vi "Main Controls.vi"() -> ()   [LabVIEW 2024]
panel:
  out "connection information":path
  out "System Number":string
  out "Idle Time":timestamp
  in  "Remove Positions":bool
  in  "Transfer Board":bool
  in  "System Summary":bool
  in  "Add Positions":bool
  in  "Exit":bool
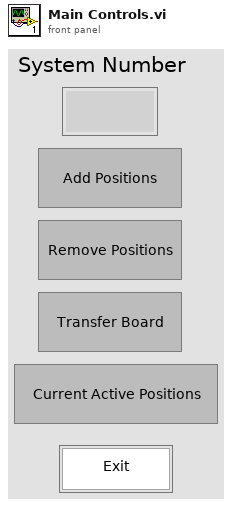
[diagram p1: front panel]
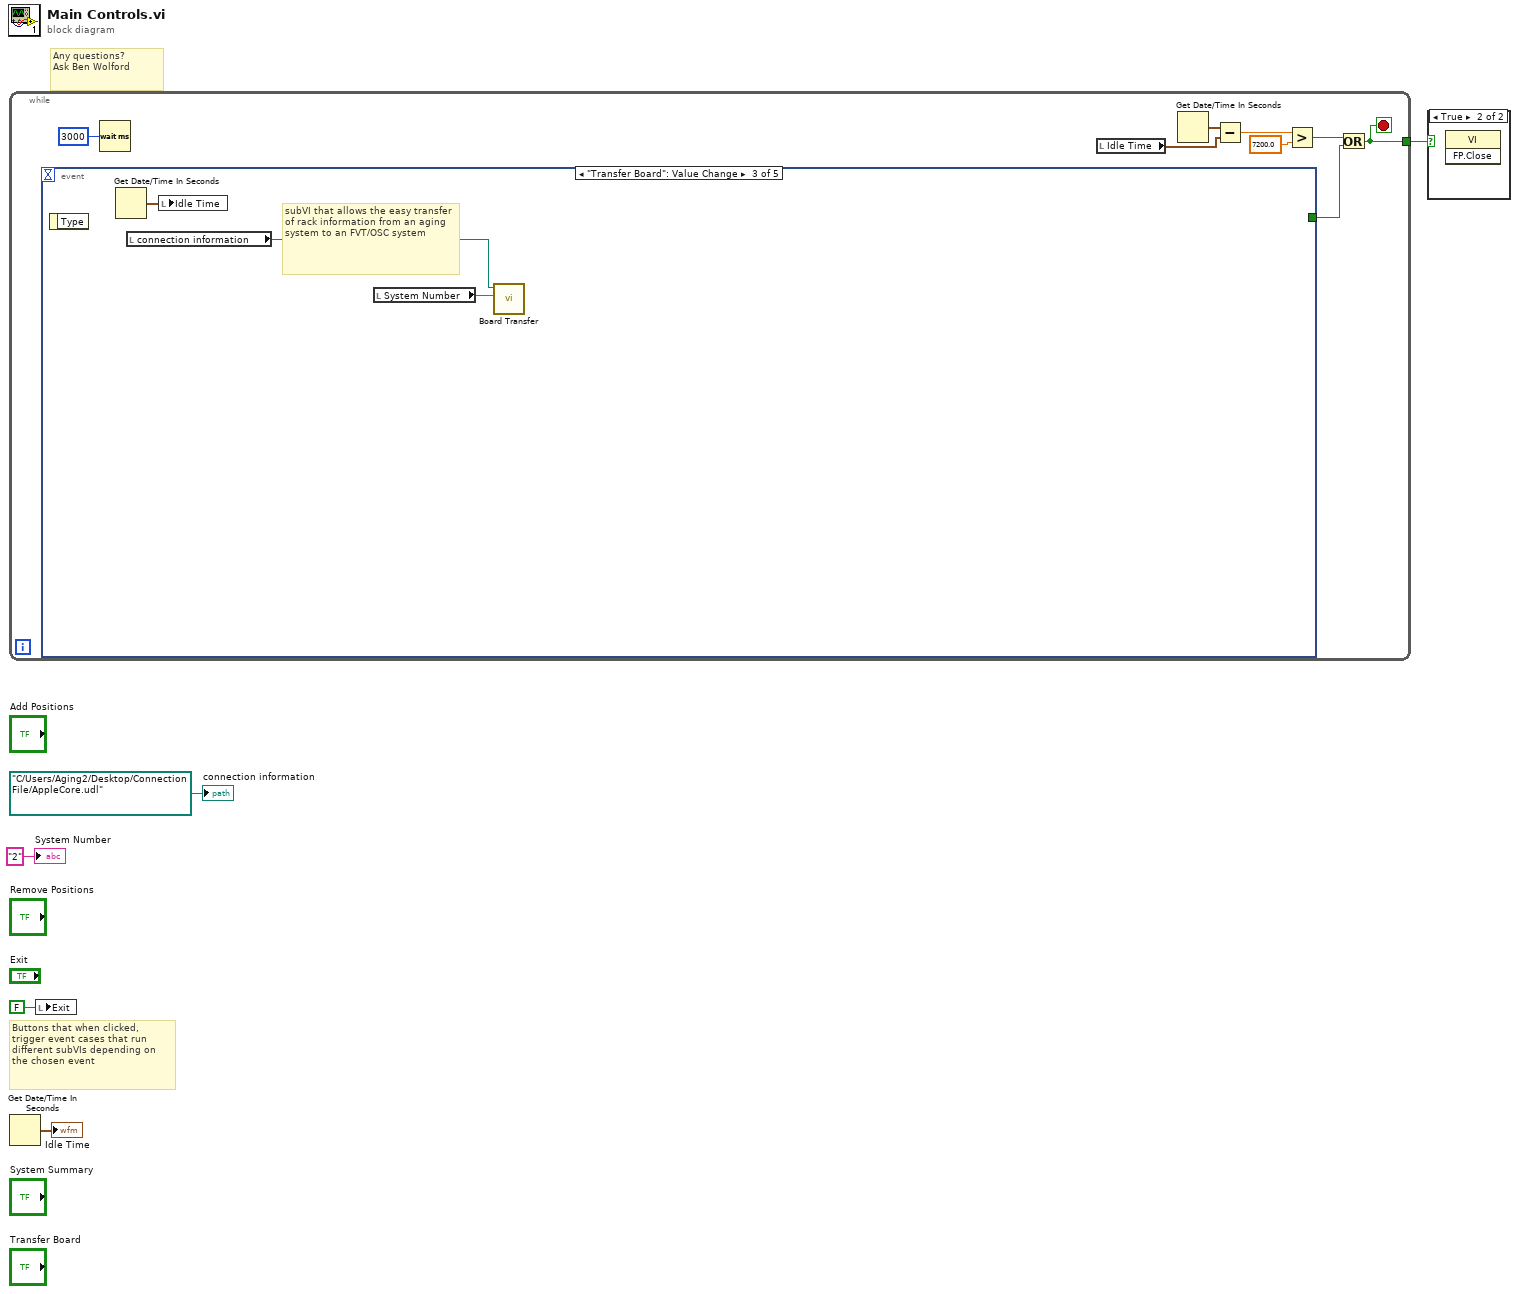
[diagram p0: block diagram]
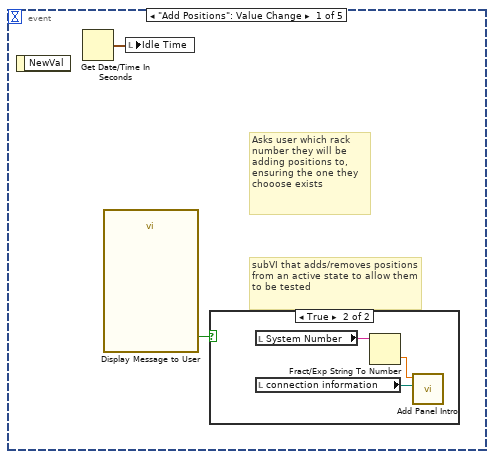
[diagram p3: hidden frame]
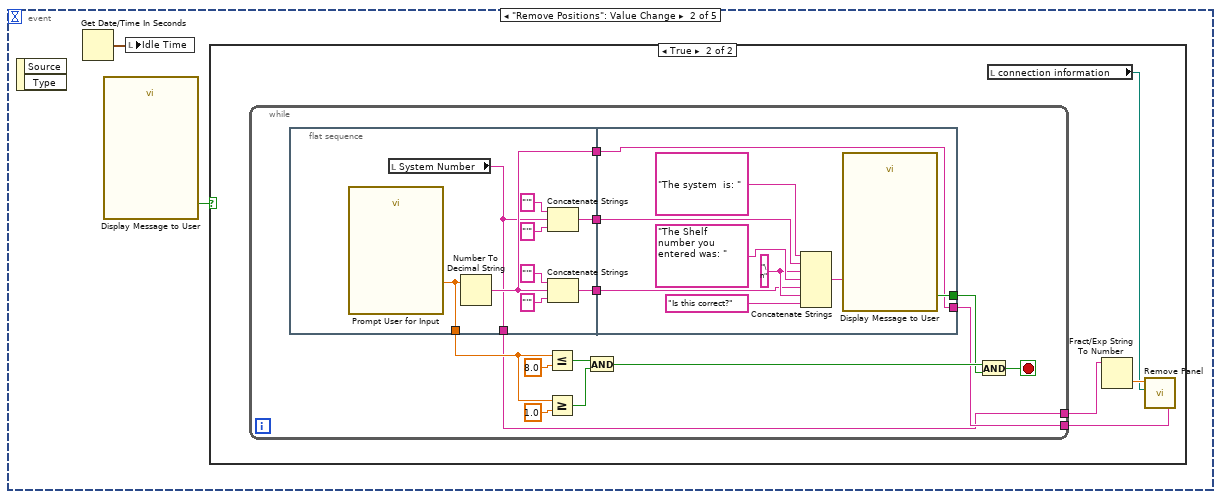
[diagram p5: hidden frame]
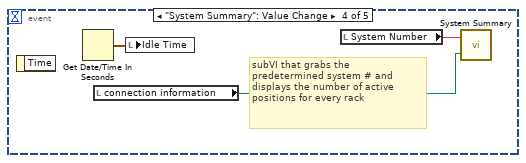
[diagram p7: hidden frame]
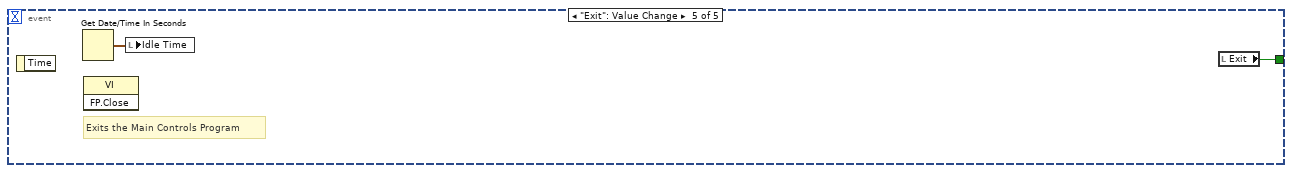
[diagram p8: hidden frame]
diagram:
  # "Buttons that when clicked, trigger event cases that run different subVIs depending on the chosen event"
  # "Any questions?\nAsk Ben Wolford"
  n1 = while {
    tunnel: [w6] -> w1
    stop <- w6 stop-if-true
    n2 = event shown="[2] \"Transfer Board\": Value Change" {
      selector: _ -> [_ _ _ _ _]
      dyn-events: _ -> [_ _ _ _ _]
      timeout: _ -> [_ _ _ _ _]
      tunnel: [_ _ _ _ w63] -> w12
      event "Add Positions": Value Change {
        # "Asks user which rack number they will be adding positions to, ensuring the one they chooose exists"
        # "subVI that adds/removes positions from an active state to allow them to be tested"
        n3 = event-data() -> ()  [unwired: 1 in, 1 out]
        n4 = Get Date/Time In Seconds() -> (seconds since 1Jan1904=w14:timestamp)
        n5 = call "Display Message to User"() -> ("Yes"=w15:bool)  [unwired: 10 in, 1 out]
        n6 = local write "Idle Time"(w14) -> ()
        n7 = case shown="True" w15 {
          frame False {
          }
          frame True {
            n8 = local read "System Number"() -> (w18:string)
            n9 = local read "connection information"() -> (w16:path)
            n10 = Fract/Exp String To Number(string=w18) -> (number=w17:dbl)  [unwired: 3 in, 1 out]
            n11 = call "Add Panel Intro.vi"("connection information"=w16, "System Number"=w17) -> ()  [unwired: 10 in]
          }
        }
      }
      event "Remove Positions": Value Change {
        n12 = event-data() -> ()  [unwired: 1 in, 2 out]
        n13 = Get Date/Time In Seconds() -> (seconds since 1Jan1904=w19:timestamp)
        n14 = call "Display Message to User"() -> ("Yes"=w20:bool)  [unwired: 10 in, 1 out]
        n15 = local write "Idle Time"(w19) -> ()
        n16 = case shown="True" w20 {
          frame False {
          }
          frame True {
            n17 = while {
              tunnel: [w26] -> w23
              tunnel: [w27] -> w24
              stop <- w29 stop-if-true
              n18 = flat-sequence {
                tunnel: [w44] -> w32
                tunnel: [w43] -> w31
                tunnel: [w40] -> w28
                tunnel: [w38] -> w26
                tunnel: [w39] -> w25
                tunnel: w32 -> [w47]
                tunnel: [w53] -> w30
                tunnel: w28 -> [w50]
                tunnel: [w48] -> w27
                tunnel: w25 -> [w48]
                frame #0 {
                  n19 = call "Prompt User for Input"() -> ("Shelf Number"=w43:dbl)  [unwired: 17 in, 2 out]
                  n20 = local read "System Number"() -> (w38:string)
                  n21 = Number To Decimal String(number=w43) -> (decimal integer string=w39:string)  [unwired: 1 in]
                  n22 = Concatenate Strings("'" ("string"), w38, "'" ("string")) -> (w40:string)
                  n23 = Concatenate Strings("'" ("string"), w39, "'" ("string")) -> (w44:string)
                }
                frame #1 {
                  w51 = "\n" ("string")
                  n24 = Concatenate Strings("The system  is: " ("string"), w50, w51, "The Shelf number you entered was: " ("string"), w47, w51, "Is this correct?" ("string")) -> (w54:string)
                  n25 = call "Display Message to User"("Message"=w54) -> ("Yes"=w53:bool)  [unwired: 9 in, 1 out]
                }
              }
              n26 = Less Or Equal?(x=w31, y=8.0) -> (x <= y?=w36:bool)
              n27 = Greater Or Equal?(x=w31, y=1.0) -> (x >= y?=w37:bool)
              n28 = And(x=w36, y=w37) -> (x .and. y?=w33:bool)
              n29 = And(x=w33, y=w30) -> (x .and. y?=w29:bool)
            }
            n30 = local read "connection information"() -> (w21:path)
            n31 = Fract/Exp String To Number(string=w23) -> (number=w22:dbl)  [unwired: 3 in, 1 out]
            n32 = call "Remove Panel.vi"("Shelf Number"=w24, "connection information"=w21, "System Num"=w22) -> ()  [unwired: 5 in]
          }
        }
      }
      event "Transfer Board": Value Change {
        # "subVI that allows the easy transfer of rack information from an aging system to an FVT/OSC system"
        n33 = event-data() -> ()  [unwired: 1 in, 1 out]
        n34 = Get Date/Time In Seconds() -> (seconds since 1Jan1904=w58:timestamp)
        n35 = local read "connection information"() -> (w57:path)
        n36 = local write "Idle Time"(w58) -> ()
        n37 = local read "System Number"() -> (w56:string)
        n38 = call "Board Transfer.vi"("SystemNumber"=w56, "connection information"=w57) -> ()  [unwired: 10 in]
      }
      event "System Summary": Value Change {
        # "subVI that grabs the predetermined system # and displays the number of active positions for every rack"
        n39 = event-data() -> ()  [unwired: 1 in, 1 out]
        n40 = Get Date/Time In Seconds() -> (seconds since 1Jan1904=w60:timestamp)
        n41 = local read "connection information"() -> (w59:path)
        n42 = local write "Idle Time"(w60) -> ()
        n43 = local read "System Number"() -> (w61:string)
        n44 = call "System Summary.vi"("connection information"=w59, "System Number"=w61) -> ()  [unwired: 1 in]
      }
      event "Exit": Value Change {
        # "Exits the Main Controls Program"
        n45 = event-data() -> ()  [unwired: 1 in, 1 out]
        n46 = Get Date/Time In Seconds() -> (seconds since 1Jan1904=w62:timestamp)
        n47 = invoke class="VI" method="FP.Close"() -> ()  [unwired: 3 in, 3 out]
        n48 = local write "Idle Time"(w62) -> ()
        n49 = local read "Exit"() -> (w63:bool)
      }
    }
    n50 = Wait (ms)(milliseconds to wait=u32 3000) -> ()  [unwired: 1 out]
    n51 = local read "Idle Time"() -> (w9:timestamp)
    n52 = Get Date/Time In Seconds() -> (seconds since 1Jan1904=w8:timestamp)
    n53 = Subtract(x=w8, y=w9) -> (x-y=w11:dbl)
    n54 = Greater?(x=w11, y=7200.0) -> (0:w7:bool)
    n55 = Or(x=w7, y=w12) -> (x .or. y?=w6:bool)
  }
  n56 = Get Date/Time In Seconds() -> (seconds since 1Jan1904=→"Idle Time":timestamp)
  n57 = local write "Exit"(FALSE ("Exit")) -> ()
  n58 = case shown="True" w1 {
    frame False {
    }
    frame True {
      n59 = invoke class="VI" method="FP.Close"() -> ()  [unwired: 3 in, 3 out]
    }
  }
  "System Number" <- "2" ("SystemNumber")
  "connection information" <- path "C:/Users/Aging2/Desktop/Connection File/AppleCore.udl" ("connection information")
